vi "Format Call Chain.vi"(7 "Call Chain":string[](array[string]), 8 "error in (no error)":errorcluster, 11 "Application Log in":refnum<class "Application Log.lvclass">) -> (0 "error out":errorcluster, 3 "Application Log out":refnum<class "Application Log.lvclass">, 4 "Formatted Call Chain":string)   [LabVIEW 2016, in "Stream Log.lvlib" / "Application Log.lvclass"]
doc: "--\nCopyright © 2017 Composed SystemsI All rights reserved.\n\nAuthor: Jon McBee <jon.mcbee@composed.io>\n\nThis library is provided \"AS IS\" ,WITHOUT WARRANTIES OR\nCONDITIONS OF ANY KIND, either express or implied.\n\nComposed Systems -- composed.io\n\nStream 0.0.1.1\nJon McBee - Composed Systems\nCopyright (c) 2017, Composed Systems"
uses:
  <userlib>/Composed Systems/Stream/Log/Application Log/Application Log.lvclass
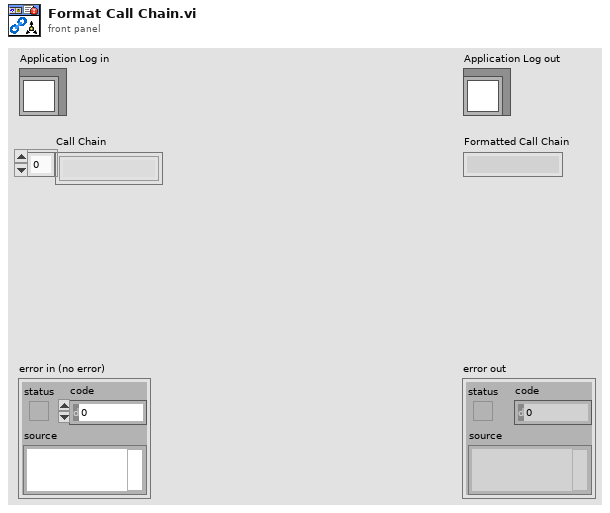
[diagram p1: front panel]
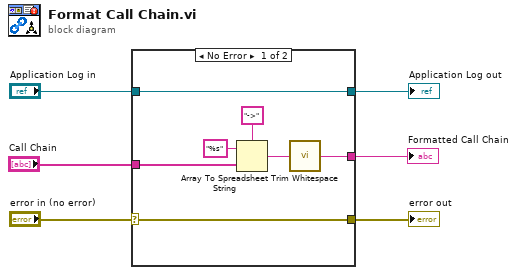
[diagram p0: block diagram]
diagram:
  n1 = case shown="No Error" "error in (no error)" {
    selector: "error in (no error)" -> [w13 w15]
    tunnel: [w13 w15] -> w5
    tunnel: [w8 w14] -> w3
    tunnel: "Application Log in" -> [w8 w14]
    tunnel: "Call Chain" -> [w12 _]
    tunnel: [w7 _] -> w1
    frame No Error {
      n2 = Array To Spreadsheet String(delimiter (Tab)="->", array=w12, 3:"%s" ("format string")) -> (spreadsheet string=w9:string)
      n3 = call <vilib>:"Trim Whitespace.vi"("string"=w9) -> ("trimmed string"=w7:string)  [unwired: 1 in]
    }
    frame Error {
    }
  }
  "error out" <- w5
  "Application Log out" <- w3
  "Formatted Call Chain" <- w1
